vi "Configure Function.vi"(8 "error in (no error)":errorcluster, 10 "Select Function (0)":i8(ring) items=["Frequency A", "Frequency B", "Frequency C", "Period", "Total", "Ratio", "T.I"], 11 "VISA resource name":refnum<visa-resource-name>) -> (0 "error out":errorcluster, 3 "VISA resource name out":refnum<visa-resource-name>)   [LabVIEW 2019, in "BK Precision 1823A.lvlib"]
doc: "This VI selects the function of the counter for display measurement. It can select between Frequency A, B, C, period, total, ratio, and T.I (Time Interval). To set to Frequency A, input integer value 0 in <b>Select Function</b>. For Frequency B, input integer 1. For Frequency C, input integer 2. For Period, 3. Total, 4. Ratio, 5. T.I, 6."
uses:
  BK Precision 1823A.lvlib
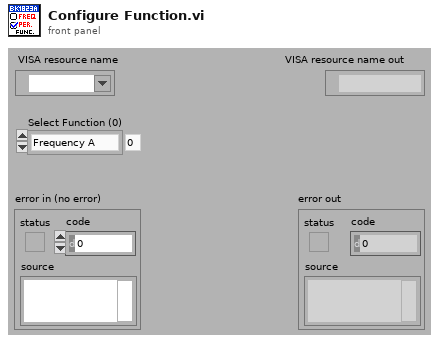
[diagram p1: front panel]
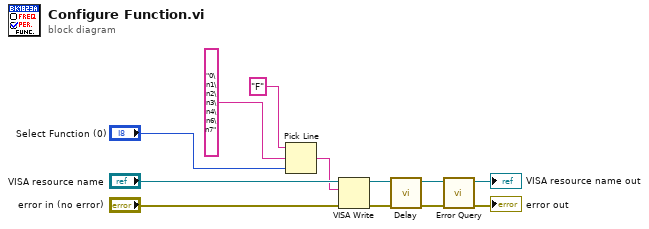
[diagram p0: block diagram]
diagram:
  n1 = Pick Line(string ("")="F", multi-line string="0\n1\n2\n3\n4\n6\n7", line index="Select Function (0)") -> (output string=w6:string)
  n2 = VISA Write(VISA resource name="VISA resource name", write buffer=w6, error in (no error)="error in (no error)") -> (VISA resource name out=w4:refnum<visa-resource-name>, error out=w3:errorcluster)  [unwired: 1 out]
  n3 = call "Delay.vi"("error in (no error)"=w3, "VISA resource name"=w4) -> ("error out"=w1:errorcluster, "VISA resource name out"=w2:refnum<visa-resource-name>)  [unwired: 8 in]
  n4 = call "Error Query.vi"("error in (no error)"=w1, "VISA resource name"=w2) -> ("error out"=→"error out":errorcluster, "VISA resource name out"=→"VISA resource name out":refnum<visa-resource-name>)  [unwired: 8 in]
